vi "DecodifyFrequency(Single).vi"(1 "32bit integer":u32) -> (0 "Frequency In":dbl=60.0 min=60.0 max=90.0 step=0.1)   [LabVIEW 2017, in "AODControl.lvlib"]
uses:
  AODControl.lvlib
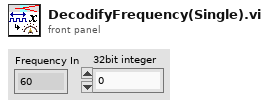
[diagram p1: front panel]
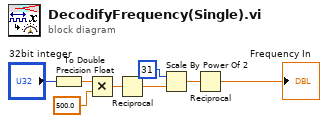
[diagram p0: block diagram]
diagram:
  n1 = To Double Precision Float(number="32bit integer") -> (double precision float=w5:dbl)
  n2 = Multiply(x=w5, y=500.0) -> (x*y=w4:dbl)
  n3 = Reciprocal(x=w4) -> (1/x=w3:dbl)
  n4 = Scale By Power Of 2(n=i16 31, x=w3) -> (x*2^n=w2:dbl)
  n5 = Reciprocal(x=w2) -> (1/x=→"Frequency In":dbl)
